vi "Read Schedule File.vi"(8 "error in (no error)":errorcluster) -> (0 "error out":errorcluster, 3 "meal schedule":T1[](array[typedef]))   [LabVIEW 2019, in "Pet Feeder.lvlib"]
uses:
  Pet Feeder.lvlib
  Controls/Feeder Program.ctl
  <vilib>/Utility/config.llb/Read Key (String).vi
  <vilib>/Utility/config.llb/Read Key (I32).vi
  <vilib>/Utility/config.llb/NI_LVConfig.lvlib
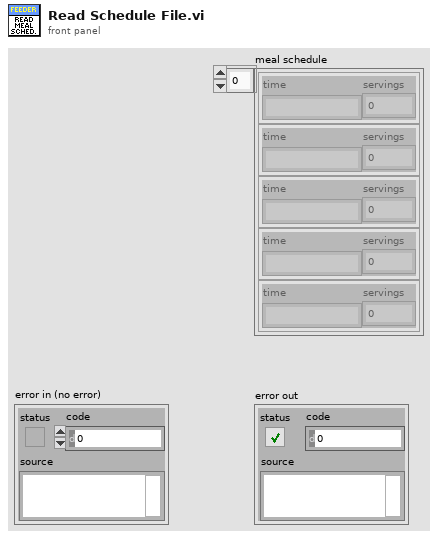
[diagram p1: front panel]
types:
  T1 = typedef "Pet Feeder.lvlib/Feeder Program.ctl" = cluster{"time":string, "servings":i32}
  T2 = typedef "NI_LVConfig.lvlib/Config Data RefNum.ctl" = refnum<k1>
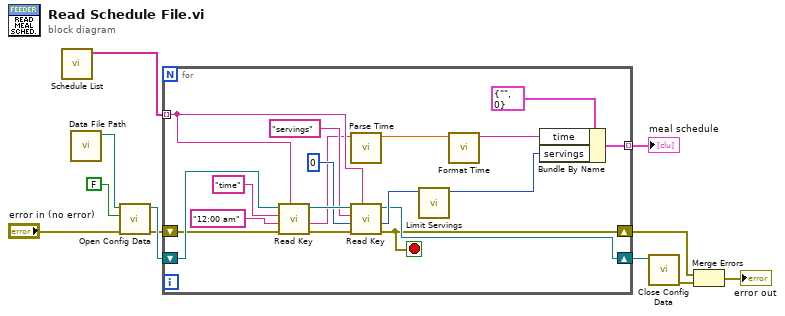
[diagram p0: block diagram]
diagram:
  n1 = call "Schedule List.vi"() -> ("schedules"=w8:string[])  [unwired: 11 in]
  n2 = call "Data File Path.vi"() -> ("data file path"=w11:path)  [unwired: 11 in]
  n3 = call <vilib>:"Open Config Data.vi"("error in (no error)"="error in (no error)", "create file if necessary (T)"=FALSE, "configuration file path"=w11) -> ("error out"=w6:errorcluster, "refnum"=w7:T2)  [unwired: 6 in, 1 out]
  n4 = for {
    tunnel: w8 -> [w24] mode=indexing
    shift-right: [w16] -> w5
    shift-left: w7 -> [w29]
    shift-right: [w15] -> w4
    shift-left: w6 -> [w26]
    tunnel: [w17] -> w1 mode=indexing
    stop <- w15 stop-if-true
    n5 = call-poly <vilib>:"Read Key.vi"("section"=w24, "error in (no error)"=w26, "default value"="12:00 am", "key"="time", "refnum"=w29) -> ("error out"=w21:errorcluster, "value"=w14:string, "refnum out"=w25:T2)  [unwired: 3 in, 1 out]
    n6 = call "Parse Time.vi"("parse time"=w14) -> ("time (HH:MM:SS)"=w13:dbl)  [unwired: 10 in]
    n7 = call-poly <vilib>:"Read Key.vi"("section"=w24, "error in (no error)"=w21, "default value"=0, "key"="servings", "refnum"=w25) -> ("error out"=w15:errorcluster, "value"=w20:i32, "refnum out"=w16:T2)  [unwired: 3 in, 1 out]
    n8 = call "Limit Servings.vi"("servings"=w20) -> ("coerced"=w18:i32)  [unwired: 10 in]
    n9 = call "Format Time.vi"("time (HH:MM:SS)"=w13) -> ("time string"=w12:string)  [unwired: 10 in]
    n10 = Bundle By Name(cluster=T1 {"time"="", "servings"=0} ("Cluster"), "time"=w12, "servings"=w18) -> (w17:T1)
  }
  "meal schedule" <- w1
  n11 = call <vilib>:"Close Config Data.vi"("refnum"=w5) -> ("error out"=w3:errorcluster)  [unwired: 9 in, 1 out]
  n12 = Merge Errors(w4, w3) -> (→"error out":errorcluster)
